vi "receive_photon_buffer.vi"(8 "error in (no error)":errorcluster, 11 "detector in":refnum<class "detector.lvclass">) -> (0 "error out":errorcluster, 2 "done":bool, 3 "detector out":refnum<class "detector.lvclass">)   [LabVIEW 2015, in "detector.lvclass"]
uses:
  detector.lvclass
  detector.lvclass/detector.ctl
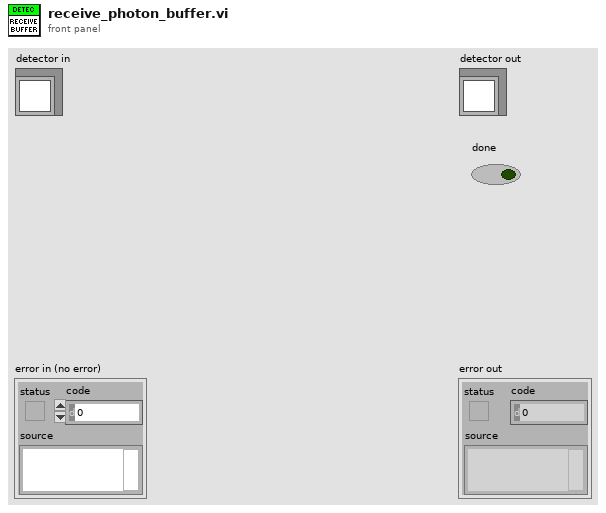
[diagram p1: front panel]
types:
  T1 = cluster{"stream":u64[], "channel":u8[], "sync":u64[], bool}
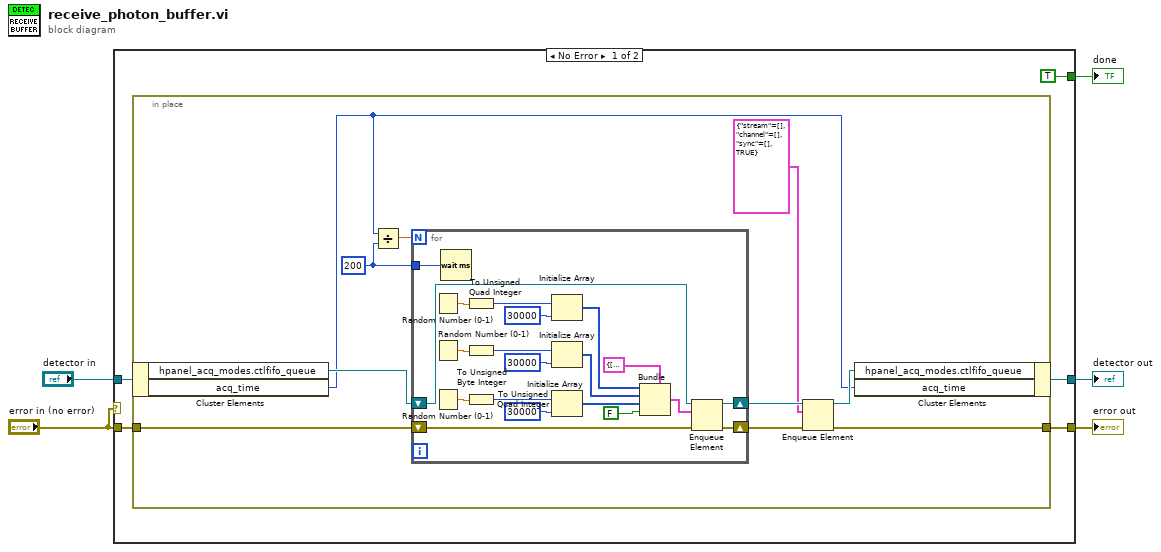
[diagram p0: block diagram]
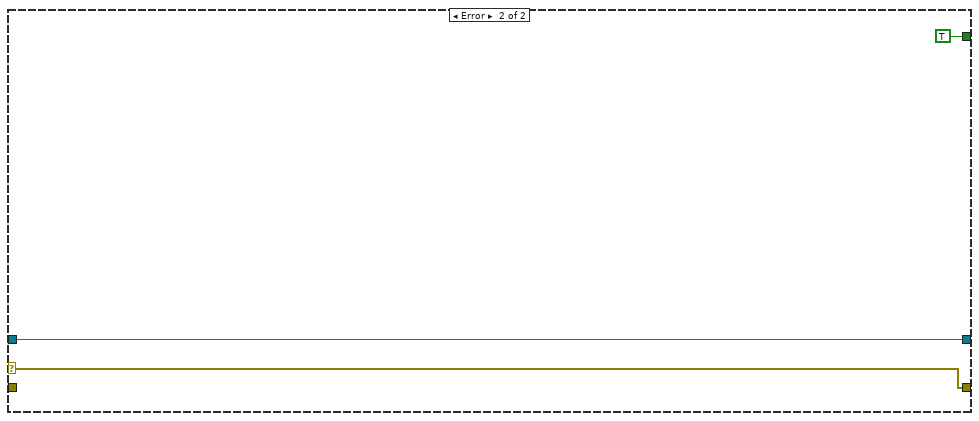
[diagram p2: hidden frame]
diagram:
  n1 = case shown="No Error" "error in (no error)" {
    selector: "error in (no error)" -> [_ w43]
    tunnel: [w7 w43] -> w5
    tunnel: [w6 w42] -> w3
    tunnel: "detector in" -> [w9 w42]
    tunnel: [TRUE ("done") TRUE ("done")] -> w2
    tunnel: "error in (no error)" -> [w8 _]
    frame No Error {
      n2 = in-place {
        in-place-border: w8 -> [w14]
        in-place-border: [w13] -> w7
        w18 = 200 ("y")
        n3 = in-place-cluster #1(w9) -> ("hpanel_acq_modes.ctlfifo_queue"=w19:refnum<queue>, "acq_time"=w11:i32)
        n4 = Divide(x=w11, y=w18) -> (x/y=w20:dbl)
        n5 = for {
          N: w20 -> [_]
          tunnel: w18 -> [w40]
          shift-right: [w32] -> w17
          shift-left: w19 -> [w39]
          shift-right: [w31] -> w15
          shift-left: w14 -> [w30]
          n6 = Random Number (0-1)() -> (number: 0 to 1=w38:dbl)
          n7 = Random Number (0-1)() -> (number: 0 to 1=w36:dbl)
          n8 = Random Number (0-1)() -> (number: 0 to 1=w37:dbl)
          n9 = Wait (ms)(milliseconds to wait=w40) -> ()  [unwired: 1 out]
          n10 = To Unsigned Quad Integer(1:w38) -> (0:w29:u64)
          n11 = To Unsigned Byte Integer(number=w36) -> (unsigned 8bit integer=w26:u8)
          n12 = To Unsigned Quad Integer(1:w37) -> (0:w22:u64)
          n13 = Initialize Array(w29, 30000 ("dimension size")) -> (w27:u64[])
          n14 = Initialize Array(w26, 30000 ("dimension size")) -> (w24:u8[])
          n15 = Initialize Array(w22, 30000 ("dimension size")) -> (w21:u64[])
          n16 = Bundle(cluster=T1 {"stream"=[], "channel"=[], "sync"=[], FALSE} ("element"), "stream"=w27, "channel"=w24, "sync"=w21, FALSE) -> (w33:T1)
          n17 = Enqueue Element(queue=w39, element=w33, error in (no error)=w30) -> (queue out=w32:refnum<queue>, error out=w31:errorcluster)  [unwired: 1 in, 1 out]
        }
        n18 = Enqueue Element(queue=w17, element=T1 {"stream"=[], "channel"=[], "sync"=[], TRUE}, error in (no error)=w15) -> (queue out=w12:refnum<queue>, error out=w13:errorcluster)  [unwired: 1 in, 1 out]
        n19 = in-place-cluster #1("hpanel_acq_modes.ctlfifo_queue"=w12, "acq_time"=w11) -> (w6:refnum<class "detector.lvclass">)
      }
    }
    frame Error {
    }
  }
  "error out" <- w5
  "detector out" <- w3
  "done" <- w2
